vi "Close Filled Text Fields.vi"(8 "error in (no error)":errorcluster, 11 "Filled Text Fields in":refnum<class "Filled Text Fields.lvclass">) -> (0 "error out":errorcluster)   [LabVIEW 2017, in "Filled Text Fields.lvlib" / "Filled Text Fields.lvclass"]
uses:
  Filled Text Fields.lvclass
  Filled Text Fields.lvclass/Filled Text Fields.ctl
  <vilib>/ActorFramework/Message Enqueuer/Message Enqueuer.lvclass/Message Enqueuer.ctl
  <vilib>/ActorFramework/Message Enqueuer/Enqueue.vi
  <vilib>/ActorFramework/Stop Msg/Stop Msg.lvclass
  C:/Program Files (x86)/National Instruments/LabVIEW 2017/vi.lib/ActorFramework/Message/Message.lvclass
  <vilib>/ActorFramework/Message Priority Queue/Priority Enqueue.vi
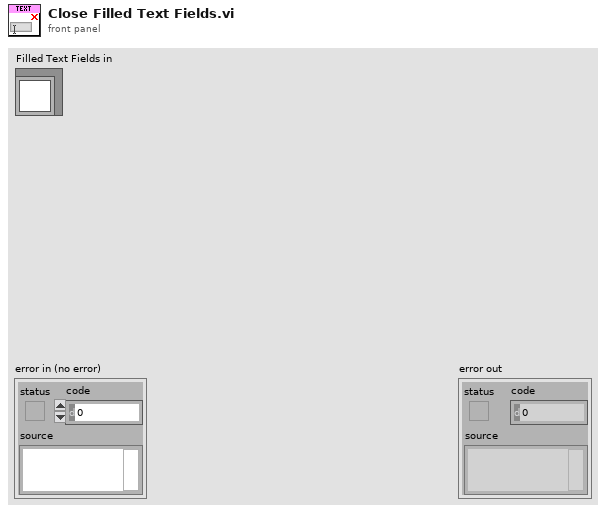
[diagram p1: front panel]
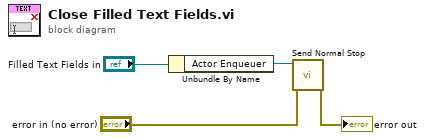
[diagram p0: block diagram]
diagram:
  n1 = Unbundle By Name("Filled Text Fields in") -> ("Actor Enqueuer"=w3:refnum<class "Message Enqueuer.lvclass">)
  n2 = call <vilib>:"Send Normal Stop.vi"("error in (no error)"="error in (no error)", "Message Enqueuer"=w3) -> ("error out"=→"error out":errorcluster)  [unwired: 9 in]
